vi "float_switch_check_debug.vi"(0 "Temperature Refnum":refnum<vi>, 1 "Heater Refnum":refnum<vi>, 2 "Abs Pressure Refnum":refnum<vi>, 3 "InvertLines":bool, 4 "Abs Temperature Limit Refnum":refnum<vi>, 5 "Timeout Refnum":refnum<vi>, 6 "Abs Pressure Limit Refnum":refnum<vi>, 7 "STOP! Refnum":refnum<vi>, 8 "Pulse Generator Slide Refnum":refnum<vi>, 9 "Float Indicator Refnum":refnum<vi>[](array[refnum]), 10 "lines array":tag[](array[tag])) -> ()   [LabVIEW 2017]
uses:
  <vilib>/DAQmx/read.llb/DAQmx Read (Digital 1D Bool NChan 1Samp 1Line).vi
  <vilib>/DAQmx/create/channels.llb/DAQmx Create Channel (DI-Digital Input).vi
  <vilib>/DAQmx/miscellaneous.llb/DAQmx Fill In Error Info.vi
  <resource>/objmgr/daqmx.rc
panel:
  out "Numeric":i32
  out "Stopwatch Elapsed":dbl
  out "Stopwatch Start":dbl
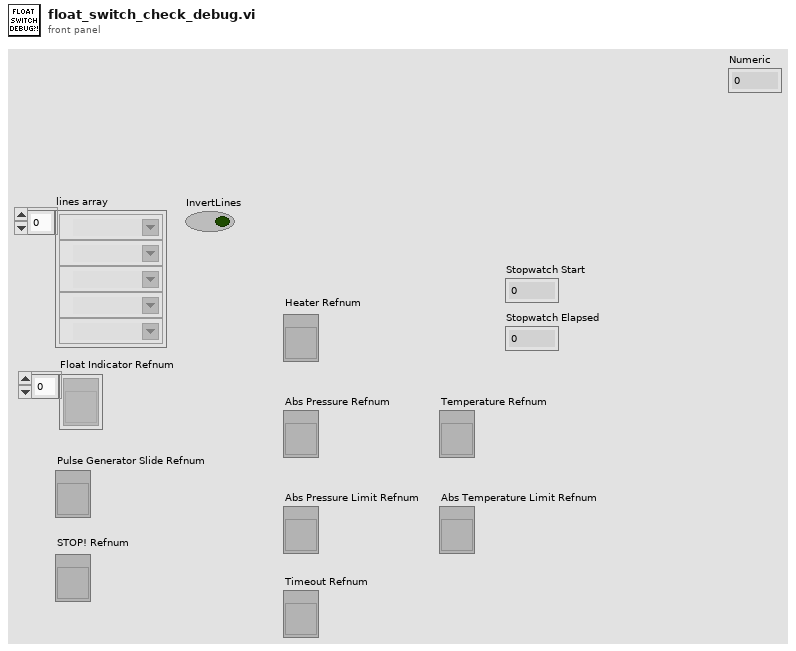
[diagram p1: front panel]
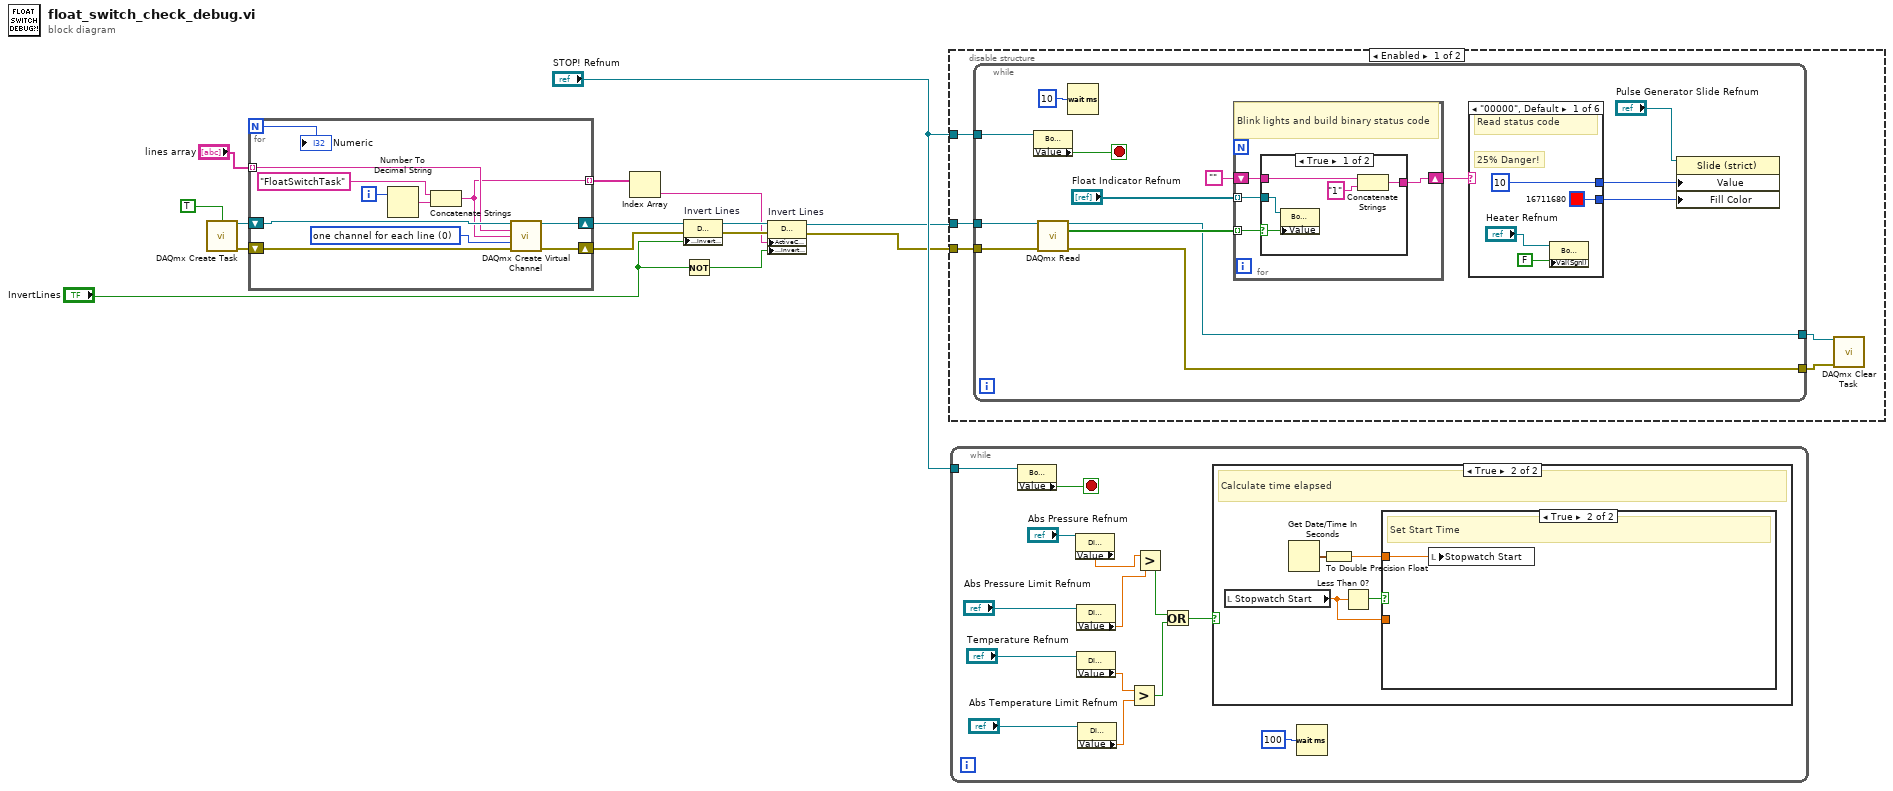
[diagram p0: block diagram]
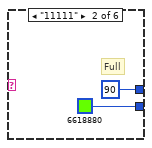
[diagram p2: hidden frame]
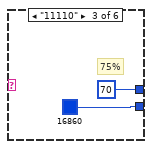
[diagram p3: hidden frame]
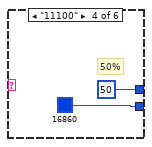
[diagram p4: hidden frame]
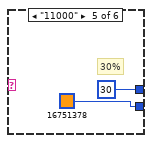
[diagram p5: hidden frame]
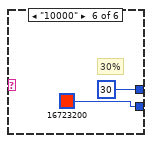
[diagram p6: hidden frame]
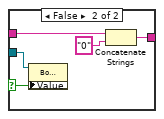
[diagram p7: hidden frame]
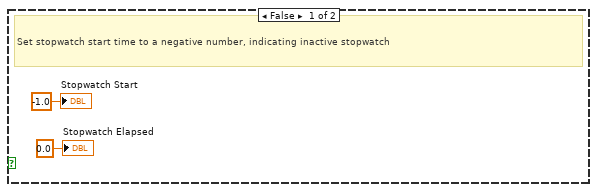
[diagram p9: hidden frame]
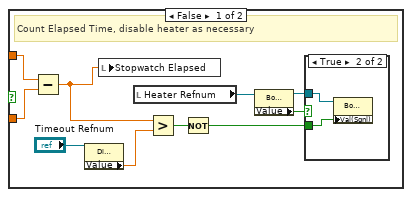
[diagram p10: hidden frame]
diagram:
  n1 = call <vilib>:"DAQmx Create Task.vi"("auto cleanup"=TRUE) -> ("task out"=w14:refnum<k21>, "error out"=w13:errorcluster)  [unwired: 13 in]
  n2 = for {
    N -> [w18]
    shift-right: [w26] -> w11
    shift-left: w14 -> [w24]
    shift-right: [w25] -> w10
    shift-left: w13 -> [w23]
    tunnel: "lines array" -> [w22] mode=indexing
    tunnel: [w16] -> w2 mode=indexing
    i -> [w19]
    w20 = 0 items=["one channel for each line", "one channel for all lines"] ("line grouping")
    n3 = Number To Decimal String(number=w19) -> (decimal integer string=w21:string)  [unwired: 1 in]
    n4 = Concatenate Strings("FloatSwitchTask" ("string"), w21) -> (w16:string)
    n5 = call-poly <vilib>:"DAQmx Create Virtual Channel.vi"("task in"=w24, "lines"=w22, "name to assign"=w16, "line grouping"=w20, "error in"=w23) -> ("task out"=w26:refnum<k21>, "error out"=w25:errorcluster)  [unwired: 9 in]
    "Numeric" <- w18
  }
  n6 = Index Array(array=w2) -> (element=w1:string)  [unwired: 1 in]
  n7 = property on="Invert Lines" class="DAQmx Channel"(reference=w11, error in=w10, "DI.InvertLines"="InvertLines") -> (reference out=w8:refnum<k21>, error out=w7:errorcluster)
  n8 = Not(x="InvertLines") -> (.not. x?=w3:bool)
  n9 = property on="Invert Lines" class="DAQmx Channel"(reference=w8, error in=w7, "ActiveChans"=w1, "DI.InvertLines"=w3) -> (reference out=w6:refnum<k21>, error out=w5:errorcluster)
  n10 = disable-structure shown="Enabled" {
    disable-tunnel: w6 -> [w31 _]
    disable-tunnel: w5 -> [w30 _]
    disable-tunnel: "STOP! Refnum" -> [w27 _]
    frame Enabled {
      n11 = while {
        tunnel: w31 -> [w40]
        tunnel: w30 -> [w39]
        tunnel: w27 -> [w35]
        tunnel: [w33] -> w29
        tunnel: [w32] -> w28
        stop <- w34 stop-if-true
        n12 = property class="Bool (strict)"(reference=w35) -> ("Value"=w34:bool)  [unwired: 1 in, 2 out]
        n13 = call-poly <vilib>:"DAQmx Read.vi"("task/channels in"=w40, "error in"=w39) -> ("task out"=w33:refnum<k21>, "data"=w45:bool[], "error out"=w32:errorcluster)  [unwired: 11 in]
        n14 = Wait (ms)(milliseconds to wait=u32 10) -> ()  [unwired: 1 out]
        n15 = for {
          tunnel: w45 -> [w63] mode=indexing
          tunnel: "Float Indicator Refnum" -> [w62] mode=indexing
          shift-right: [w60] -> w43
          shift-left: "" -> [w61]
          # "Blink lights and build binary status code"
          n16 = case shown="True" w63 {
            selector: w63 -> [w67 w72]
            tunnel: w62 -> [w68 w73]
            tunnel: w61 -> [w66 w70]
            tunnel: [w64 w69] -> w60
            frame True {
              n17 = property class="Bool (strict)"(reference=w68, "Value"=w67) -> ()  [unwired: 1 in, 2 out]
              n18 = Concatenate Strings(w66, "1" ("string")) -> (w64:string)
            }
            frame False {
              n19 = property class="Bool (strict)"(reference=w73, "Value"=w72) -> ()  [unwired: 1 in, 2 out]
              n20 = Concatenate Strings(w70, "0" ("string")) -> (w69:string)
            }
          }
        }
        n21 = case shown="\"00000\", Default" w43 {
          tunnel: [u8 10 u8 90 u8 70 u8 50 u8 30 u8 30] -> w42
          tunnel: [u32 16711680 u32 6618880 u32 16860 u32 16860 u32 16751378 u32 16723200] -> w41
          frame "00000", Default {
            # "25% Danger!"
            # "Read status code"
            n22 = property class="Bool (strict)"(reference="Heater Refnum", "Val(Sgnl)"=FALSE) -> ()  [unwired: 1 in, 2 out]
          }
          frame "11111" {
            # "Full"
          }
          frame "11110" {
            # "75%"
          }
          frame "11100" {
            # "50%"
          }
          frame "11000" {
            # "30%"
          }
          frame "10000" {
            # "30%"
          }
        }
        n23 = property class="Slide (strict)"(reference="Pulse Generator Slide Refnum", "Value"=w42, "Fill Color"=w41) -> ()  [unwired: 1 in, 2 out]
      }
      n24 = call <vilib>:"DAQmx Clear Task.vi"("task in"=w29, "error in"=w28) -> ()  [unwired: 13 in, 1 out]
    }
    frame Disabled {
    }
  }
  n25 = while {
    tunnel: "STOP! Refnum" -> [w86]
    stop <- w87 stop-if-true
    n26 = property class="Bool (strict)"(reference=w86) -> ("Value"=w87:bool)  [unwired: 1 in, 2 out]
    n27 = property class="DigNum (strict)"(reference="Abs Pressure Refnum") -> ("Value"=w75:dbl)  [unwired: 1 in, 2 out]
    n28 = property class="DigNum (strict)"(reference="Abs Pressure Limit Refnum") -> ("Value"=w74:dbl)  [unwired: 1 in, 2 out]
    n29 = property class="DigNum (strict)"(reference="Temperature Refnum") -> ("Value"=w80:dbl)  [unwired: 1 in, 2 out]
    n30 = property class="DigNum (strict)"(reference="Abs Temperature Limit Refnum") -> ("Value"=w79:dbl)  [unwired: 1 in, 2 out]
    n31 = Greater?(x=w80, y=w79) -> (0:w77:bool)
    n32 = Greater?(x=w75, y=w74) -> (0:w78:bool)
    n33 = Or(x=w78, y=w77) -> (x .or. y?=w76:bool)
    n34 = case shown="True" w76 {
      frame False {
        # "Set stopwatch start time to a negative number, indicating inactive stopwatch"
        "Stopwatch Start" <- -1.0 ("Stopwatch Start")
        "Stopwatch Elapsed" <- 0.0 ("Stopwatch Elapsed")
      }
      frame True {
        # "Calculate time elapsed"
        n35 = local read "Stopwatch Start"() -> (w90:dbl)
        n36 = Get Date/Time In Seconds() -> (seconds since 1Jan1904=w92:timestamp)
        n37 = To Double Precision Float(number=w92) -> (double precision float=w91:dbl)
        n38 = Less Than 0?(x=w90) -> (x < 0?=w93:bool)
        n39 = case shown="True" w93 {
          tunnel: w91 -> [w103 w106]
          tunnel: w90 -> [w102 _]
          frame False {
            # "Count Elapsed Time, disable heater as necessary"
            n40 = Subtract(x=w103, y=w102) -> (x-y=w98:dbl)
            n41 = property class="DigNum (strict)"(reference="Timeout Refnum") -> ("Value"=w100:dbl)  [unwired: 1 in, 2 out]
            n42 = local write "Stopwatch Elapsed"(w98) -> ()
            n43 = local read "Heater Refnum"() -> (w97:refnum<vi>)
            n44 = Greater?(x=w98, y=w100) -> (0:w99:bool)
            n45 = Not(x=w99) -> (.not. x?=w94:bool)
            n46 = property class="Bool (strict)"(reference=w97) -> (reference out=w95:refnum<vi>, "Value"=w96:bool)  [unwired: 1 in, 1 out]
            n47 = case shown="True" w96 {
              tunnel: w95 -> [_ w105]
              tunnel: w94 -> [_ w104]
              frame False {
              }
              frame True {
                n48 = property class="Bool (strict)"(reference=w105, "Val(Sgnl)"=w104) -> ()  [unwired: 1 in, 2 out]
              }
            }
          }
          frame True {
            # "Set Start Time"
            n49 = local write "Stopwatch Start"(w106) -> ()
          }
        }
      }
    }
    n50 = Wait (ms)(milliseconds to wait=u32 100) -> ()  [unwired: 1 out]
  }
